vi "Calibrate GPS Device.vi"() -> ()   [LabVIEW 2011]
uses:
  <vilib>/Utility/file.llb/Write To Spreadsheet File (DBL).vi
panel:
  in  "Actual Longitude":dbl=-121.863188
  in  "Actual Latitude":dbl=39.736001
  out "Current Longitude":dbl format="%_13g"
  out "Current Latitude":dbl format="%_13g"
  out "Longitude Array":dbl[](array[numeric]) format="%#_11g"
  out "Latitude Array":dbl[](array[numeric]) format="%#_11g"
  out "Iteration":i32
  in  "VISA resource name":refnum<visa-resource-name>="COM3"
  out "Averaged Longitude":dbl format="%#_11g"
  out "Averaged Latitude":dbl format="%#_11g"
  out "Longitude Fluctuation Error":dbl format="%#_11g"
  out "Latitude Fluctuation Error":dbl format="%#_11g"
  out "Raw Averaged Longitude":dbl
  out "Raw Averaged Latitude":dbl
  out "Latitude Zero Error":dbl format="%#.11g"
  out "Longitude Zero Error":dbl format="%#.11g"
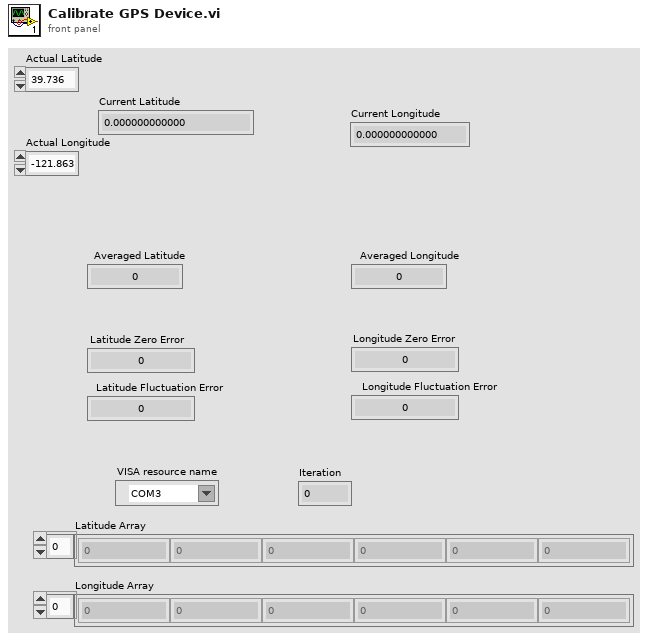
[diagram p1: front panel]
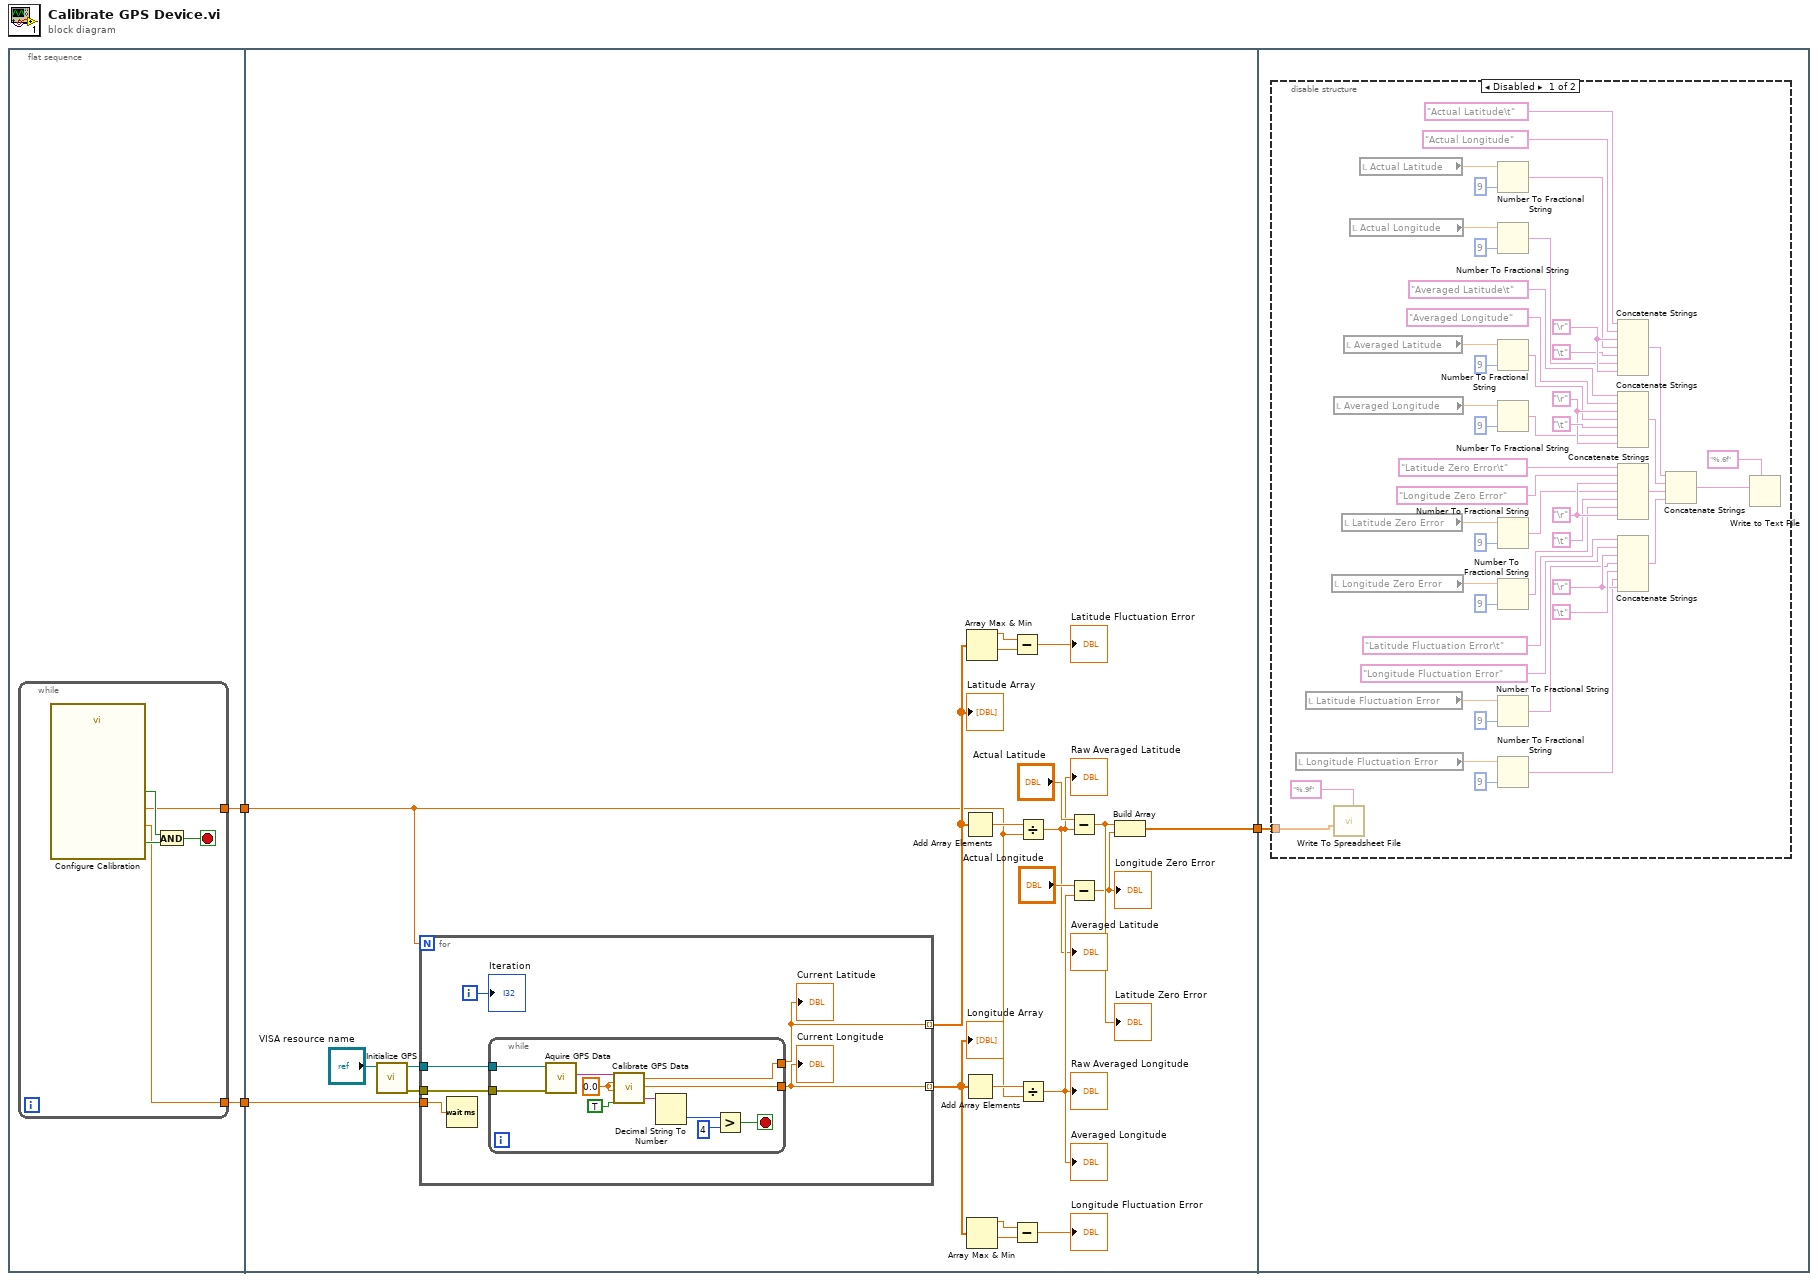
[diagram p0: block diagram]
diagram:
  n1 = flat-sequence {
    tunnel: [w5] -> w2
    tunnel: [w4] -> w1
    tunnel: [w18] -> w3
    tunnel: w2 -> [w16]
    tunnel: w1 -> [w15]
    tunnel: w3 -> [w50]
    frame #0 {
      n2 = while {
        tunnel: [w7] -> w5
        tunnel: [w6] -> w4
        stop <- w10 stop-if-true
        n3 = call "Configure Calibration"() -> ("Confirm Antenna Position"=w9:bool, "Period (ms)"=w6:dbl, "Samples"=w7:dbl, "Calibrate"=w8:bool)  [unwired: 15 in, 1 out]
        n4 = And(x=w8, y=w9) -> (x .and. y?=w10:bool)
      }
    }
    frame #1 {
      n5 = call "Initialize GPS.vi"("VISA resource name"="VISA resource name") -> ("error out"=w11:errorcluster, "VISA resource name out"=w12:refnum<visa-resource-name>)  [unwired: 9 in]
      n6 = for {
        N: w16 -> [_]
        tunnel: w11 -> [w38]
        tunnel: w12 -> [w37]
        tunnel: [w34] -> w27 mode=indexing
        tunnel: [w35] -> w28 mode=indexing
        tunnel: w15 -> [w36]
        i -> [w33]
        n7 = Wait (ms)(milliseconds to wait=w36) -> ()  [unwired: 1 out]
        n8 = while {
          tunnel: w38 -> [w49]
          tunnel: w37 -> [w48]
          tunnel: [w45] -> w35
          tunnel: [w44] -> w34
          stop <- w39 stop-if-true
          w46 = 0.0 ("Latitude Error")
          n9 = call "Aquire GPS Data.vi"("error in"=w49, "VISA resource name in"=w48) -> ("read buffer"=w47:string)  [unwired: 7 in, 2 out]
          n10 = call "Calibrate GPS Data.vi"("Read Buffer"=w47, "Latitude Error"=w46, "Longitude Error"=w46, "Calibrate"=TRUE) -> ("Latitude"=w45:dbl, "Longitude"=w44:dbl, "Satellites Tracked"=w40:string)  [unwired: 16 in, 5 out]
          n11 = Decimal String To Number(string=w40) -> (number=w41:i32)  [unwired: 2 in, 1 out]
          n12 = Greater?(x=w41, y=4) -> (0:w39:bool)
        }
        "Current Latitude" <- w35
        "Current Longitude" <- w34
        "Iteration" <- w33
      }
      "Latitude Array" <- w28
      "Longitude Array" <- w27
      n13 = Add Array Elements(numeric array=w28) -> (sum=w30:dbl)
      n14 = Add Array Elements(numeric array=w27) -> (sum=w29:dbl)
      n15 = Array Max & Min(array=w28) -> (max value=w26:dbl, min value=w25:dbl)  [unwired: 2 out]
      n16 = Array Max & Min(array=w27) -> (max value=w24:dbl, min value=w23:dbl)  [unwired: 2 out]
      n17 = Subtract(x=w26, y=w25) -> (x-y=→"Latitude Fluctuation Error":dbl)
      n18 = Subtract(x=w24, y=w23) -> (x-y=→"Longitude Fluctuation Error":dbl)
      n19 = Divide(x=w30, y=w16) -> (x/y=w13:dbl)
      "Raw Averaged Latitude" <- w13
      "Averaged Latitude" <- w13
      n20 = Divide(x=w29, y=w16) -> (x/y=w14:dbl)
      "Raw Averaged Longitude" <- w14
      "Averaged Longitude" <- w14
      n21 = Subtract(x="Actual Latitude", y=w13) -> (x-y=w20:dbl)
      "Latitude Zero Error" <- w20
      n22 = Subtract(x="Actual Longitude", y=w14) -> (x-y=w19:dbl)
      "Longitude Zero Error" <- w19
      n23 = Build Array(w20, w19) -> (w18:dbl[])
    }
    frame #2 {
      n24 = disable-structure shown="Disabled" {
        disable-tunnel: w50 -> [w98 _]
        frame Disabled {
          w82 = "\r"
          w83 = "\r"
          w90 = "\r"
          w92 = "\r"
          n25 = local read "Longitude Fluctuation Error"() -> (w59:dbl)
          n26 = local read "Latitude Fluctuation Error"() -> (w60:dbl)
          n27 = local read "Longitude Zero Error"() -> (w57:dbl)
          n28 = local read "Averaged Longitude"() -> (w72:dbl)
          n29 = call-poly <vilib>:"Write To Spreadsheet File.vi"("format (%.3f)"="%.9f", "1D data"=w98) -> ()  [unwired: 6 in, 1 out]
          n30 = local read "Latitude Zero Error"() -> (w58:dbl)
          n31 = local read "Averaged Latitude"() -> (w70:dbl)
          n32 = local read "Actual Longitude"() -> (w61:dbl)
          n33 = local read "Actual Latitude"() -> (w62:dbl)
          n34 = Number To Fractional String(number=w62, precision (6)=i16 9) -> (F-format string=w51:string)  [unwired: 2 in]
          n35 = Number To Fractional String(number=w61, precision (6)=i16 9) -> (F-format string=w52:string)  [unwired: 2 in]
          n36 = Number To Fractional String(number=w70, precision (6)=i16 9) -> (F-format string=w69:string)  [unwired: 2 in]
          n37 = Number To Fractional String(number=w72, precision (6)=i16 9) -> (F-format string=w71:string)  [unwired: 2 in]
          n38 = Number To Fractional String(number=w58, precision (6)=i16 9) -> (F-format string=w55:string)  [unwired: 2 in]
          n39 = Number To Fractional String(number=w57, precision (6)=i16 9) -> (F-format string=w56:string)  [unwired: 2 in]
          n40 = Number To Fractional String(number=w60, precision (6)=i16 9) -> (F-format string=w53:string)  [unwired: 2 in]
          n41 = Number To Fractional String(number=w59, precision (6)=i16 9) -> (F-format string=w54:string)  [unwired: 2 in]
          n42 = Concatenate Strings("Actual Latitude\t" ("string"), "Actual Longitude" ("string"), w90, w51, "\t", w52, w90) -> (w78:string)
          n43 = Concatenate Strings("Averaged Latitude\t" ("string"), "Averaged Longitude" ("string"), w92, w69, "\t", w71, w92) -> (w77:string)
          n44 = Concatenate Strings("Latitude Zero Error\t" ("string"), "Longitude Zero Error" ("string"), w82, w55, "\t", w56, w82) -> (w76:string)
          n45 = Concatenate Strings("Latitude Fluctuation Error\t" ("string"), "Longitude Fluctuation Error" ("string"), w83, w53, "\t", w54, w83) -> (w75:string)
          n46 = Concatenate Strings(w78, w77, w76, w75) -> (w91:string)
          n47 = Write to Text File(prompt (Choose or enter file path)="%.6f" ("format (%.3f)"), text=w91) -> ()  [unwired: 2 in, 3 out]
        }
        frame Enabled {
        }
      }
    }
  }
